vi "PLL analyzer -- PID -- V3.vi"(0 "frequency IN (Hz)":dbl=-1.0 format="%#_10f", 1 "voltage IN (V)":cdb=-0.0017981943418797428+0.0018232090265536353i format="%#_10f", 4 "time in (sec)":dbl=289.5873590533738, 5 "lorentzian IN":T2={"A (VHz)"=0.003914650866681924, "f (Hz)"=44855.11779996251, "G (Hz)"=2.9247633391664567, "phi(rad)"=3.909694945239435, "Q"=15336.32386569301, "Norm  Ampl"=nan, "bg (V)"=0.00013625172364348747-0.00019483842623467182i, "4corners"={"z (-pi/2)"=-0.0017563199699203156-0.00016210148449623068i, "z(inf)"=0.00013625172364348747-0.00019483842623467182i, "z (pi/2)"=0.0001689886653819286+0.0016977332673291314i, "z center"=-0.0007936656522691936+0.0007678158914164503i, "z(0)"=-0.0017235830281818747+0.0017304702090675725i, "radius"=0.0013384504702515796}} {"bg (V)" format="%#9_9f"; "Q" format="%#9_9f"; "phi(rad)" format="%#9_9f"; "G (Hz)" format="%#9_9f"; "f (Hz)" format="%#9_9f"}, 6 "PID action":T4, 7 "requested size":i32=100, 10 "PLL limits (Hz)":dbl=5000.0 format="%#.2f", 11 "PID mode":T1, 12 "dt (sec)":dbl=0.02 format="%#_10f", 13 "PID parameters":T5={"I (sec)"=4.747474747474747, "P (sec)"=2.0765656565656565} {"P (sec)" scale=0.01..10.0; "I (sec)" scale=0.01..10.0}) -> (14 "frequency OUT (Hz)":dbl=-1.0 format="%#_10f", 15 "overlimit ?":bool=TRUE, 18 "time out (sec)":dbl=289.5873590533738, 19 "lorentzian  OUT":T2={"A (VHz)"=0.003914650866681924, "f (Hz)"=44855.11779996251, "G (Hz)"=2.9247633391664567, "phi(rad)"=3.909694945239435, "Q"=15336.32386569301, "Norm  Ampl"=nan, "bg (V)"=0.00013625172364348747-0.00019483842623467182i, "4corners"={"z (-pi/2)"=-0.0017563199699203156-0.00016210148449623068i, "z(inf)"=0.00013625172364348747-0.00019483842623467182i, "z (pi/2)"=0.0001689886653819286+0.0016977332673291314i, "z center"=-0.0007936656522691936+0.0007678158914164503i, "z(0)"=-0.0017235830281818747+0.0017304702090675725i, "radius"=0.0013384504702515796}} {"bg (V)" format="%#9_9f"; "Q" format="%#9_9f"; "phi(rad)" format="%#9_9f"; "G (Hz)" format="%#9_9f"; "f (Hz)" format="%#9_9f"})   [LabVIEW 2020]
uses:
  pid -- parameters.ctl
  PID action.ctl
  lorentzian.ctl
  circle corners.ctl
  PID - mode.ctl
  agregator -- action.ctl
  four-corner circle transformation.ctl
  Q - not nan -- real.vi
  linear interpolation iiii- complex.vi
  linear interpolation - real.vi
panel:
  out "Plot: complex plane":cluster{dbl[], dbl[]}[](graph)=[{[], []}, {[nan, nan, nan, nan, nan, nan, nan, nan, nan, nan, nan, nan, nan, nan, nan, nan, nan, nan, nan, nan, nan, nan, nan, nan, nan, nan, nan, nan, nan, nan, nan, nan, nan, nan, nan, nan, nan, nan, nan, nan, nan, nan, nan, nan, nan, nan, nan, nan, nan, nan], [nan, nan, nan, nan, nan, nan, nan, nan, nan, nan, nan, nan, nan, nan, nan, nan, nan, nan, nan, nan, nan, nan, nan, nan, nan, nan, nan, nan, nan, nan, nan, nan, nan, nan, nan, nan, nan, nan, nan, nan, nan, nan, nan, nan, nan, nan, nan, nan, nan, nan]}, {[nan, nan, nan, nan, nan, nan, nan, nan, nan, nan, nan, nan, nan, nan, nan, nan, nan, nan, nan, nan], [nan, nan, nan, nan, nan, nan, nan, nan, nan, nan, nan, nan, nan, nan, nan, nan, nan, nan, nan, nan]}, {[nan, nan, nan, nan, nan, nan, nan, nan, nan, nan, nan, nan, nan, nan, nan, nan, nan, nan, nan, nan], [nan, nan, nan, nan, nan, nan, nan, nan, nan, nan, nan, nan, nan, nan, nan, nan, nan, nan, nan, nan]}, {[nan, nan, nan, nan, nan, nan, nan, nan, nan, nan, nan, nan, nan, nan, nan, nan, nan, nan, nan, nan], [nan, nan, nan, nan, nan, nan, nan, nan, nan, nan, nan, nan, nan, nan, nan, nan, nan, nan, nan, nan]}, {[nan, nan, nan, nan, nan, nan, nan, nan, nan, nan, nan, nan, nan, nan, nan, nan, nan, nan, nan, nan], [nan, nan, nan, nan, nan, nan, nan, nan, nan, nan, nan, nan, nan, nan, nan, nan, nan, nan, nan, nan]}, {[], []}]
  in  "Plot: complex plane - filter":cluster{dbl[], dbl[]}[](graph)=[{[], []}, {[], []}, {[0.0, 0.0, 0.0, 0.0, 0.0, 0.0, 0.0, 0.0, 0.0, 0.0, 0.0, 0.0, 0.0, 0.0, 0.0, 0.0, 0.0, 0.0, 0.0, 0.0, 0.0, 0.0, 0.0, 0.0, 0.0, 0.0, 0.0, 0.0, 0.0, 0.0, 0.0, 0.0, 0.0, 0.0, 0.0, 0.0, 0.0, 0.0, 0.0, 0.0, 0.0, 0.0, 0.0, 0.0, 0.0, 0.0, 0.0, 0.0, 0.0, 0.0, 0.0, 0.0, 0.0, 0.0, 0.0, 0.0, 0.0, 0.0, 0.0, 0.0, 0.0, 0.0, 0.0, 0.0, 0.0, 0.0, 0.0, 0.0, 0.0, 0.0, 0.0, 0.0, 0.0, 0.0, 0.0, 0.0, 0.0, 0.0, 0.0, 0.0, 0.0, 0.0, 0.0, 0.0, 0.0, 0.0, 0.0, 0.0, 0.0, 0.0, 0.0, 0.0, 0.0, 0.0, 0.0, 0.0, 0.0, 0.0, 0.0, 0.0], [0.0, 0.0, 0.0, 0.0, 0.0, 0.0, 0.0, 0.0, 0.0, 0.0, 0.0, 0.0, 0.0, 0.0, 0.0, 0.0, 0.0, 0.0, 0.0, 0.0, 0.0, 0.0, 0.0, 0.0, 0.0, 0.0, 0.0, 0.0, 0.0, 0.0, 0.0, 0.0, 0.0, 0.0, 0.0, 0.0, 0.0, 0.0, 0.0, 0.0, 0.0, 0.0, 0.0, 0.0, 0.0, 0.0, 0.0, 0.0, 0.0, 0.0, 0.0, 0.0, 0.0, 0.0, 0.0, 0.0, 0.0, 0.0, 0.0, 0.0, 0.0, 0.0, 0.0, 0.0, 0.0, 0.0, 0.0, 0.0, 0.0, 0.0, 0.0, 0.0, 0.0, 0.0, 0.0, 0.0, 0.0, 0.0, 0.0, 0.0, 0.0, 0.0, 0.0, 0.0, 0.0, 0.0, 0.0, 0.0, 0.0, 0.0, 0.0, 0.0, 0.0, 0.0, 0.0, 0.0, 0.0, 0.0, 0.0, 0.0]}, {[0.0, 0.0, 0.0], [0.0, 0.0, 0.0]}, {[nan, nan, nan, nan, nan, nan, nan, nan, nan, nan, nan, nan, nan, nan, nan, nan, nan, nan, nan, nan], [nan, nan, nan, nan, nan, nan, nan, nan, nan, nan, nan, nan, nan, nan, nan, nan, nan, nan, nan, nan]}, {[0.0, 0.0, 0.0, 0.0, 0.0, 0.0, 0.0, 0.0, 0.0, 0.0, 0.0, 0.0, 0.0, 0.0, 0.0, 0.0, 0.0, 0.0, 0.0, 0.0], [0.0, 0.0, 0.0, 0.0, 0.0, 0.0, 0.0, 0.0, 0.0, 0.0, 0.0, 0.0, 0.0, 0.0, 0.0, 0.0, 0.0, 0.0, 0.0, 0.0]}]
  out "pm lorentzian":T2={"A (VHz)"=nan, "f (Hz)"=0.0, "G (Hz)"=0.0, "phi(rad)"=nan, "Q"=nan, "Norm  Ampl"=nan, "bg (V)"=nan+nani, "4corners"={"z (-pi/2)"=nan+nani, "z(inf)"=nan+nani, "z (pi/2)"=nan+nani, "z center"=nan+nani, "z(0)"=nan+nani, "radius"=nan}} {"bg (V)" format="%#9_9f"; "Q" format="%#9_9f"; "phi(rad)" format="%#9_9f"; "G (Hz)" format="%#9_9f"; "f (Hz)" format="%#9_9f"}
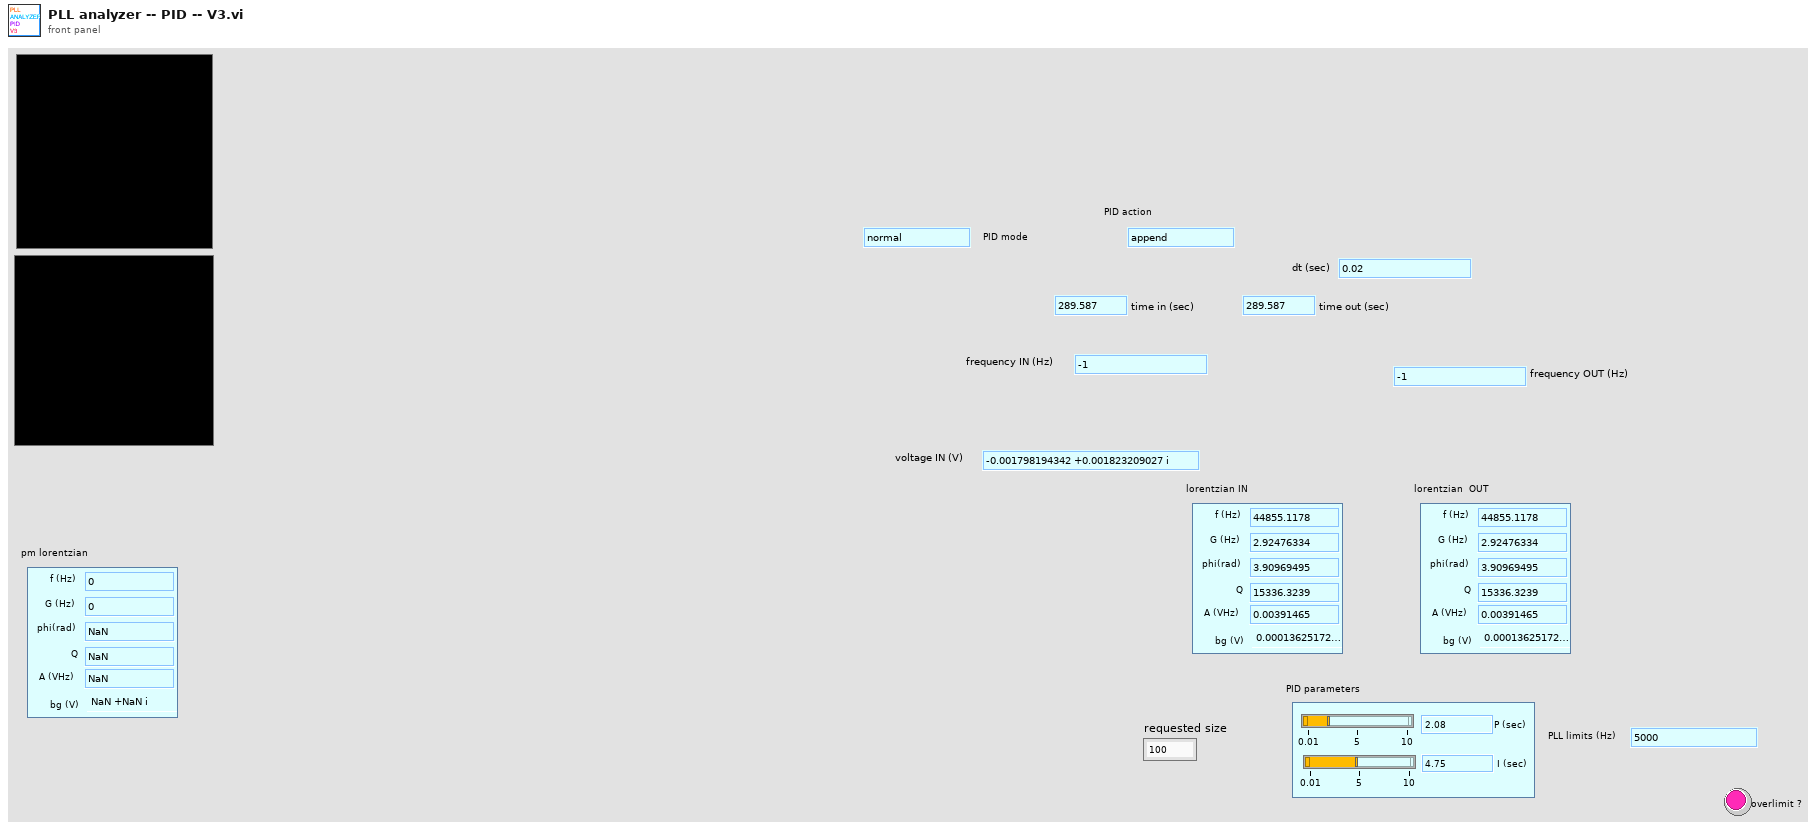
[diagram p1: front panel]
types:
  T1 = typedef "PID - mode.ctl" = enum16{"normal", "heat"}
  T2 = typedef "lorentzian.ctl" = cluster{"A (VHz)":dbl, "f (Hz)":dbl, "G (Hz)":dbl, "phi(rad)":dbl, "Q":dbl, "Norm  Ampl":dbl, "bg (V)":cdb, "4corners":T3}
  T3 = typedef "circle corners.ctl" = cluster{"z (-pi/2)":cdb, "z(inf)":cdb, "z (pi/2)":cdb, "z center":cdb, "z(0)":cdb, "radius":dbl}
  T4 = typedef "PID action.ctl" = enum16{"append", "empty!", "reset frequency", "reset from num", "overlimit"}
  T5 = typedef "pid -- parameters.ctl" = cluster{"I (sec)":dbl, "P (sec)":dbl}
  T6 = typedef "agregator -- action.ctl" = enum16{"append", "interpolate", "empty!", "force", "init", "scale", "read last"}
  T7 = typedef "four-corner circle transformation.ctl" = enum16{"z(c) z(inf)", "z(c) z(zero)", "fix phase", "calculate lorentzian", "z(0) z(+-pi/2)", "shift to zcenter", "to  canonical", "get canonical phase", "get4corners", "update lorentzian -- from z0", "fake gamma normal", "fake gamma heat", "calculate complex slope"}
  T8 = typedef "interpolation state - real.ctl" = cluster{"requested size":i32, "Array":dbl[], "actual number of elements":i32}
  T9 = typedef "interpolation state - complex.ctl" = cluster{"requested size":i32, "Array":cdb[], "actual number of elements":i32}
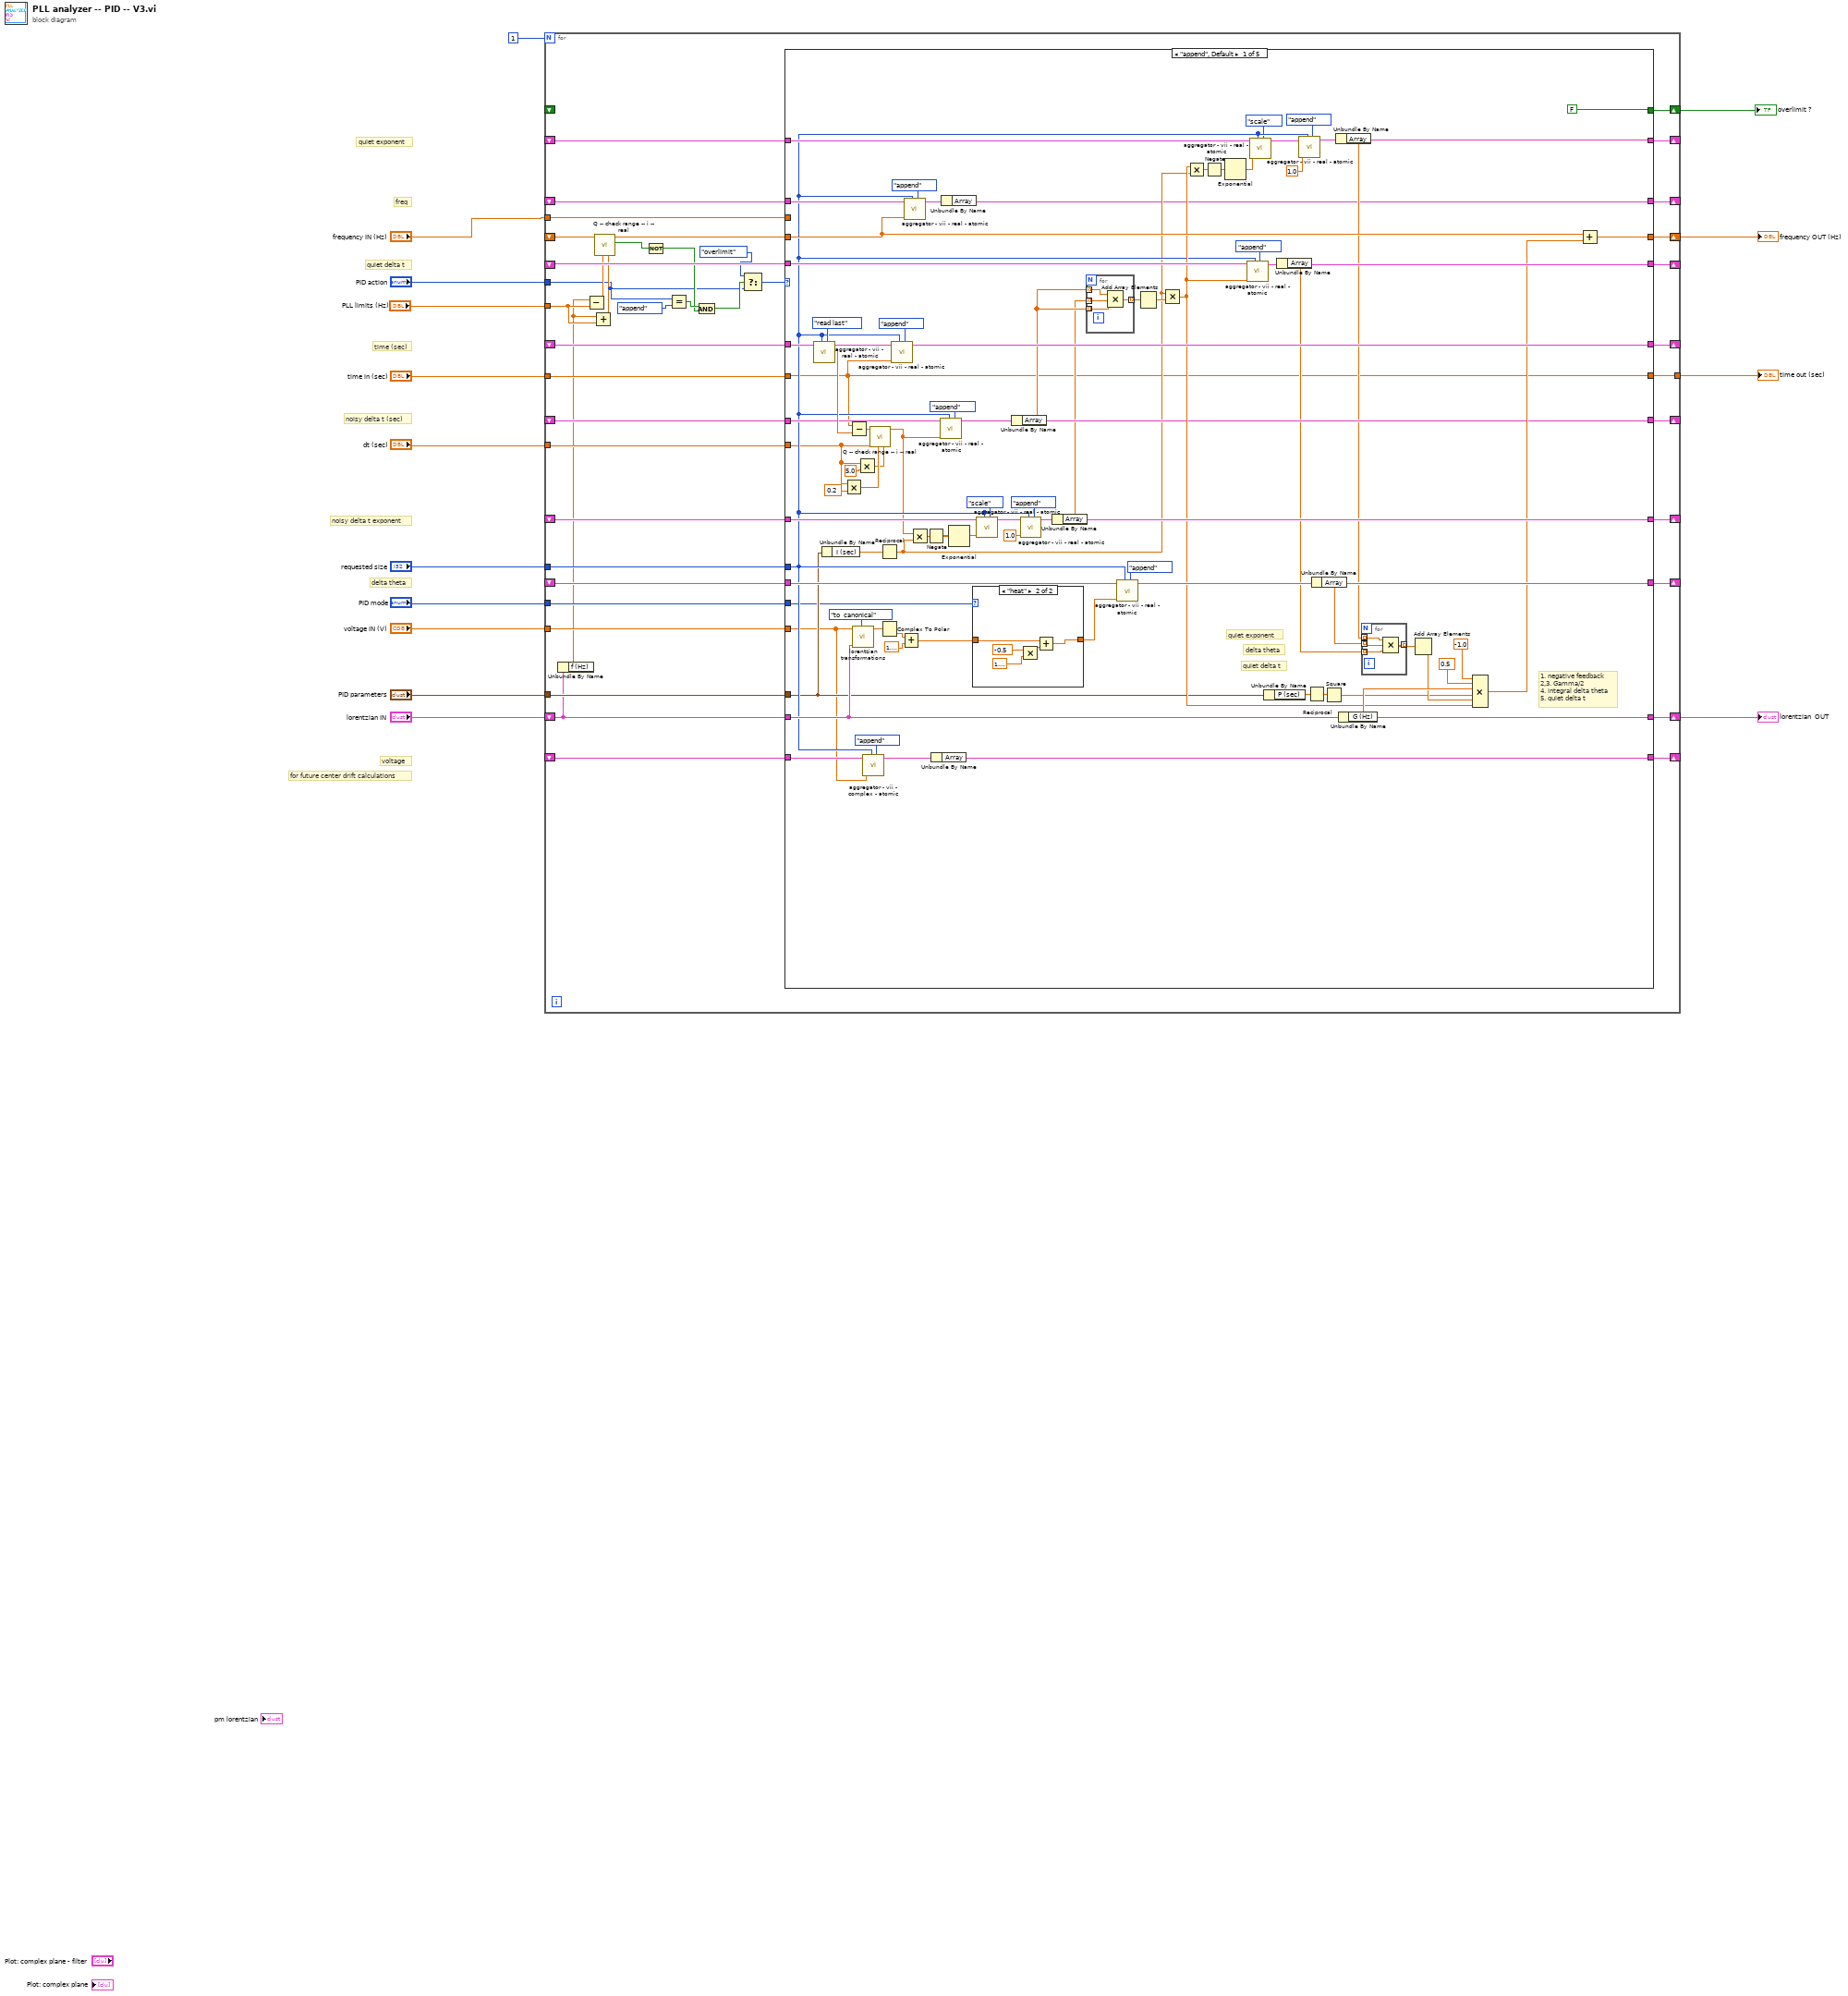
[diagram p0: block diagram]
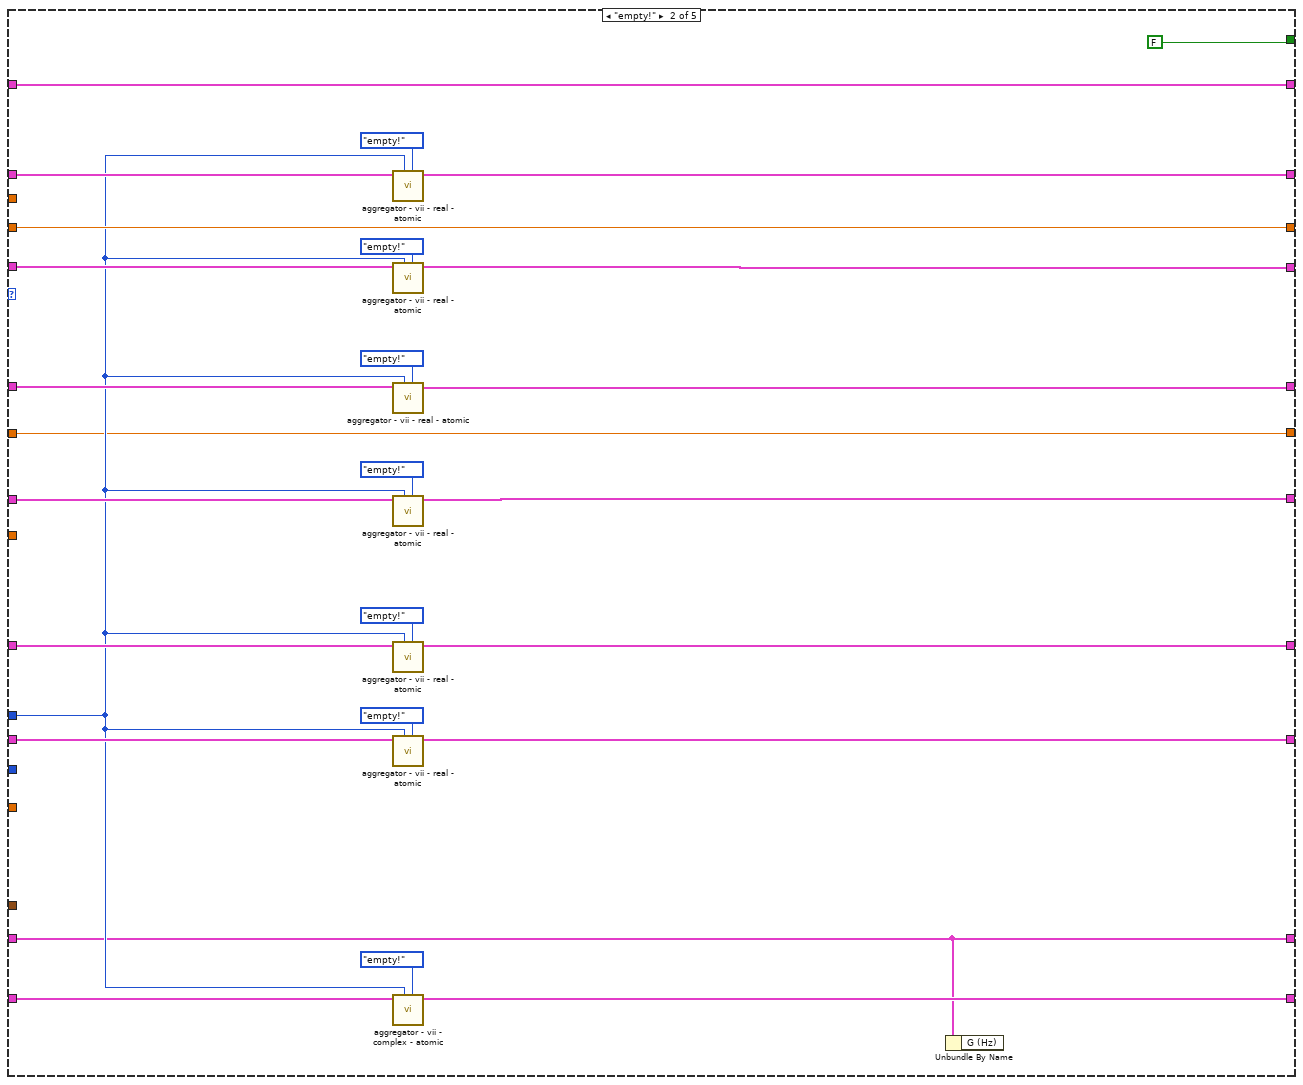
[diagram p3: hidden frame]
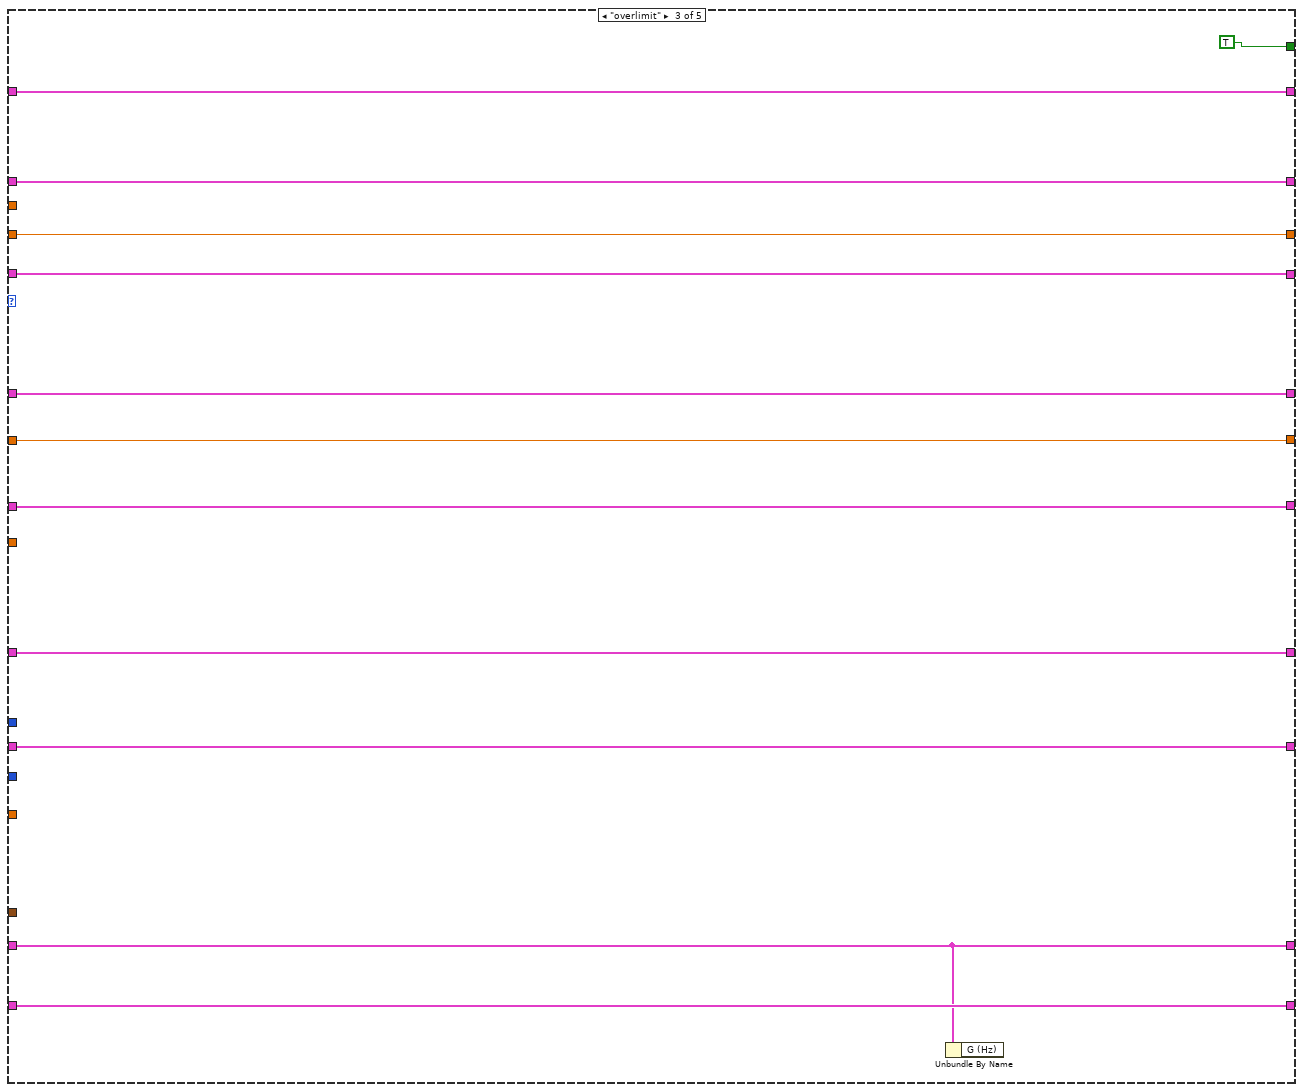
[diagram p4: hidden frame]
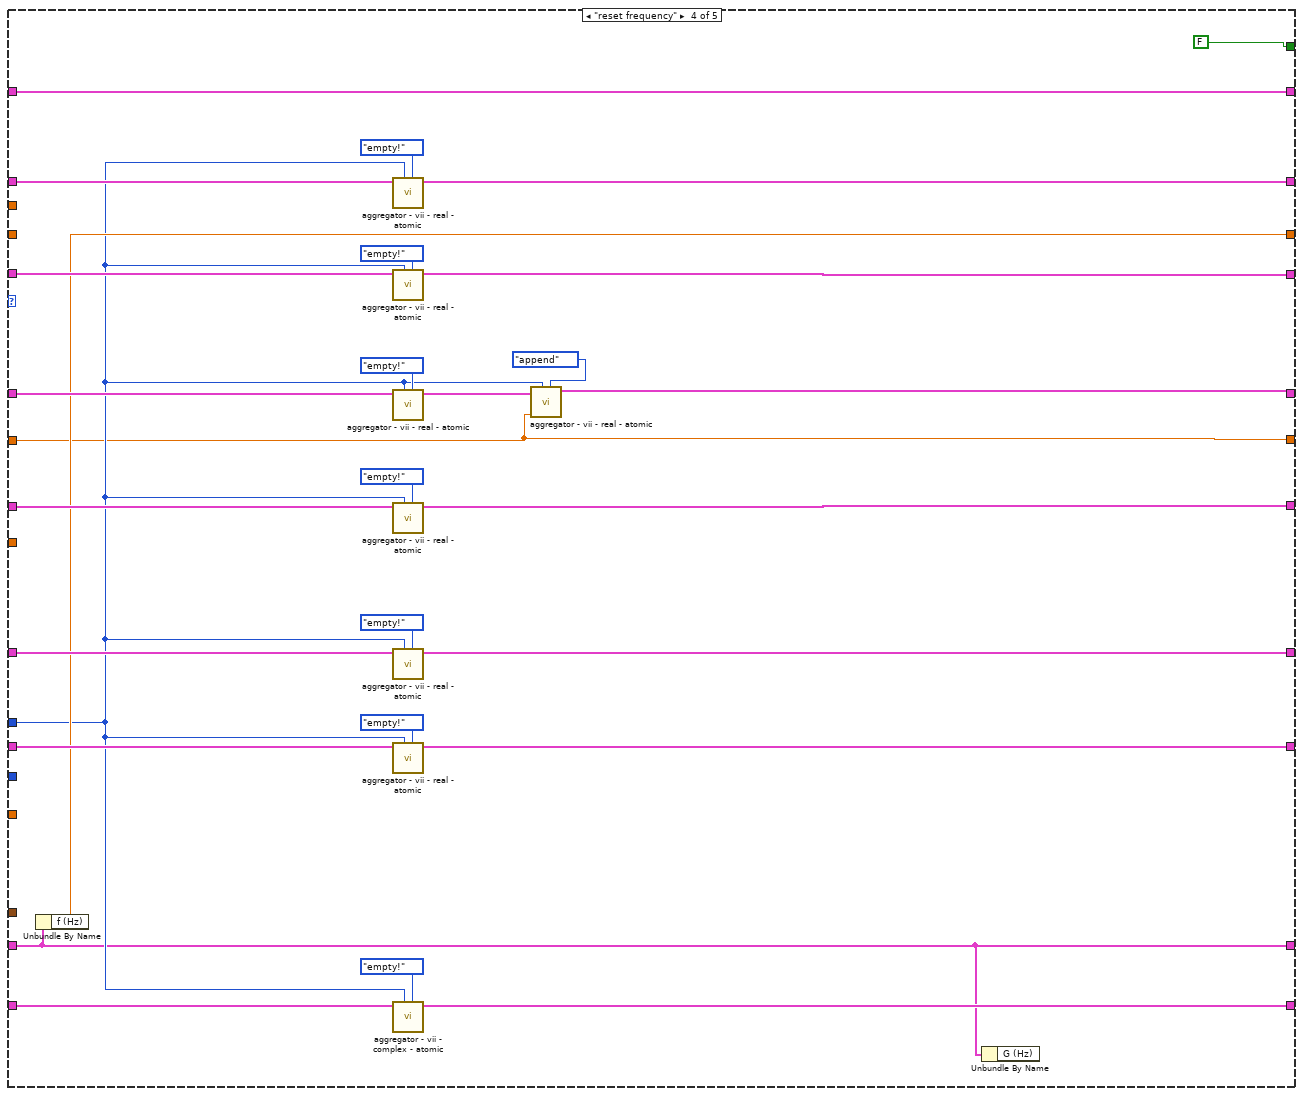
[diagram p5: hidden frame]
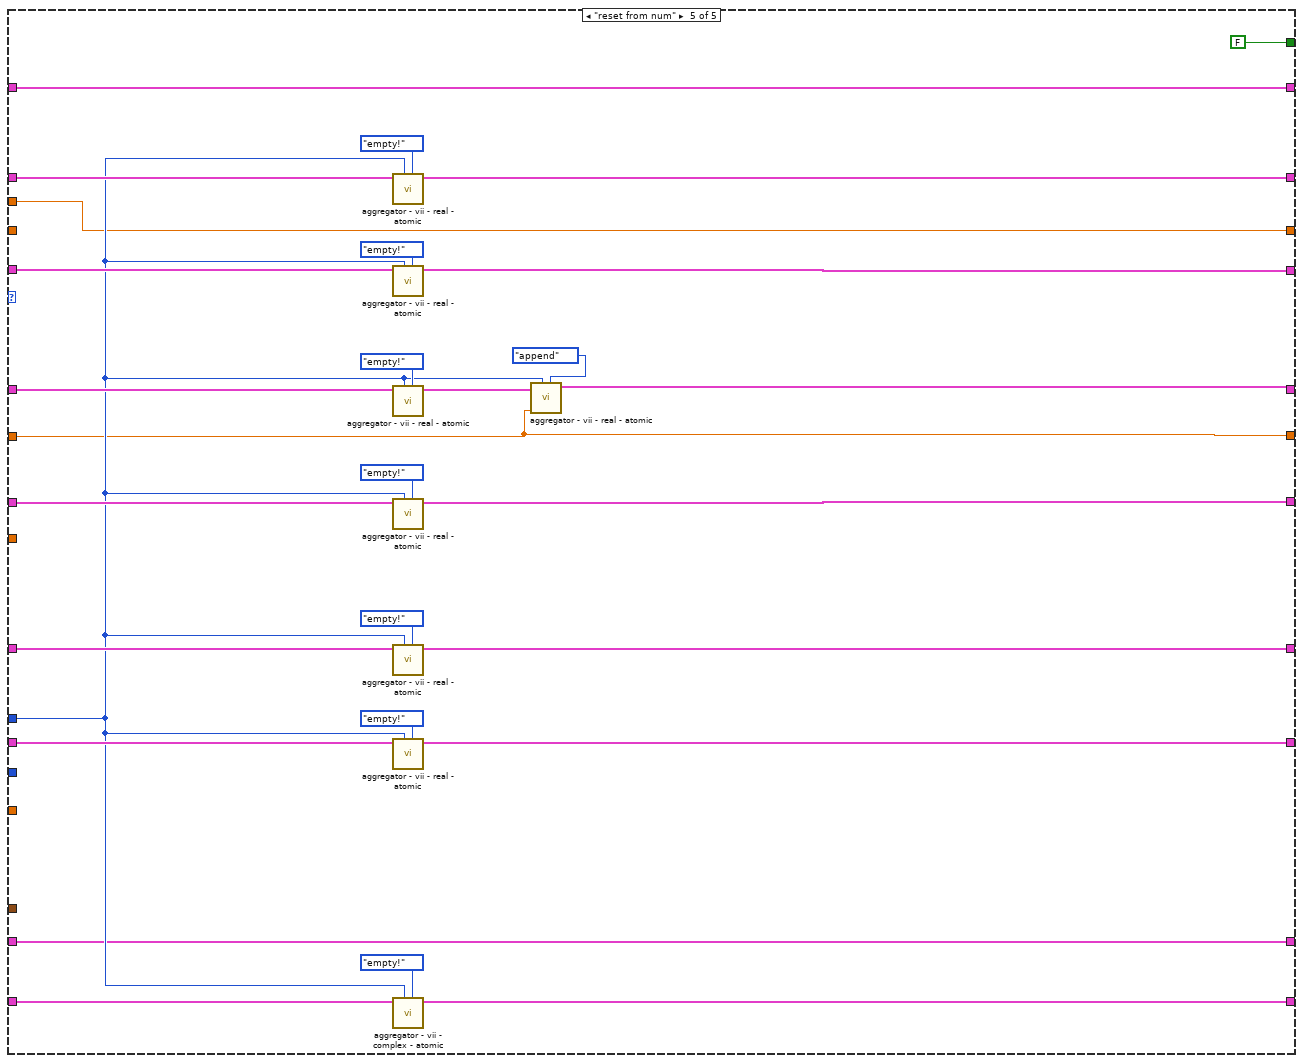
[diagram p6: hidden frame]
diagram:
  # "quiet exponent"
  # "noisy delta t exponent"
  # "for future center drift calculations"
  # "voltage"
  # "freq"
  # "delta theta"
  # "quiet delta t"
  # "time (sec)"
  # "noisy delta t (sec)"
  n1 = for {
    N: 1 -> [_]
    tunnel: "requested size" -> [w57]
    tunnel: "PID action" -> [w16]
    shift-right: [w55] -> _
    shift-left: _ -> [w56]
    tunnel: "time in (sec)" -> [w54]
    shift-right: [w52] -> _
    shift-left: _ -> [w53]
    tunnel: "voltage IN (V)" -> [w51]
    shift-right: [w49] -> _
    shift-left: _ -> [w50]
    shift-right: [w47] -> _
    shift-left: _ -> [w48]
    shift-right: [w46] -> w4
    shift-left: _ -> [w26]
    shift-right: [w45] -> w10
    shift-left: "lorentzian IN" -> [w28]
    shift-right: [w44] -> _
    shift-left: _ -> [w43]
    shift-right: [w42] -> _
    shift-left: _ -> [w41]
    shift-right: [w40] -> _
    shift-left: _ -> [w39]
    shift-right: [w38] -> _
    shift-left: _ -> [w37]
    tunnel: "frequency IN (Hz)" -> [w36]
    tunnel: "dt (sec)" -> [w35]
    tunnel: "PID parameters" -> [w34]
    tunnel: [w33] -> w6
    tunnel: "PID mode" -> [w32]
    tunnel: "PLL limits (Hz)" -> [w29]
    shift-right: [w23] -> w2
    shift-left: _ -> [_]
    n2 = Unbundle By Name(w28) -> ("f (Hz)"=w27:dbl)
    n3 = Subtract(x=w27, y=w29) -> (x-y=w31:dbl)
    n4 = Add(x=w27, y=w29) -> (x+y=w30:dbl)
    n5 = call "Q -- check range -- i -- real.vi"("upper"=w30, "lower"=w31, "number"=w26) -> ("in range?"=w20:bool, "number in range"=w25:dbl)  [unwired: 6 in, 1 out]
    n6 = Not(x=w20) -> (.not. x?=w19:bool)
    n7 = Equal?(x=w16, y=PID_action."append" ("f")) -> (x = y?=w21:bool)
    n8 = And(x=w21, y=w19) -> (x .and. y?=w18:bool)
    n9 = Select(t=PID_action."overlimit" ("f"), s=w18, f=w16) -> (s? t:f=w24:T4)
    n10 = case shown="\"append\", Default" w24 {
      tunnel: w57 -> [w95 w156 _ w195 w225]
      tunnel: w56 -> [w137 w168 w187 w209 w238]
      tunnel: [w118 w155 w187 w196 w226] -> w55
      tunnel: w54 -> [w65 w154 w181 w194 w224]
      tunnel: w53 -> [w136 w172 w189 w213 w242]
      tunnel: [w123 w171 w189 w212 w241] -> w52
      tunnel: w51 -> [w62 _ _ _ _]
      tunnel: w50 -> [w103 w170 w188 w211 w240]
      tunnel: [w90 w169 w188 w210 w239] -> w49
      tunnel: w48 -> [w127 w174 w190 w215 w244]
      tunnel: [w125 w173 w190 w214 w243] -> w47
      tunnel: w25 -> [w108 w167 w186 _ _]
      tunnel: w28 -> [w111 w153 w180 w191 w220]
      tunnel: [w120 w167 w186 w199 w222] -> w46
      tunnel: [w111 w153 w180 w191 w220] -> w45
      tunnel: [w59 w165 w185 w193 w223] -> w44
      tunnel: w43 -> [w110 w166 w185 w208 w237]
      tunnel: [w58 w161 w184 w204 w233] -> w42
      tunnel: w41 -> [w109 w162 w184 w205 w234]
      tunnel: [w92 w159 w183 w202 w231] -> w40
      tunnel: w39 -> [w100 w158 w183 w201 w230]
      tunnel: [w91 w157 w182 w200 w229] -> w38
      tunnel: w37 -> [w99 w157 w182 w200 w229]
      tunnel: w36 -> [_ _ _ _ w222]
      tunnel: w35 -> [w75 _ _ _ _]
      tunnel: w34 -> [w68 _ _ _ _]
      tunnel: [w65 w154 w181 w194 w224] -> w33
      tunnel: w32 -> [w61 _ _ _ _]
      tunnel: [FALSE FALSE TRUE FALSE FALSE] -> w23
      frame "append", Default {
        # "1. negative feedback\n2,3. Gamma/2\n4. integral delta theta\n5. quiet delta t"
        # "quiet delta t"
        # "delta theta"
        # "quiet exponent"
        n11 = call "aggregator - vii - real - atomic.vi"("aggregator action"=agregator_--_action."read last", "requested size"=w95, "state IN"=w137) -> ("mean"=w130:dbl, "state OUT"=w119:T8)  [unwired: 5 in, 2 out]
        n12 = Unbundle By Name(w68) -> ("I (sec)"=w67:dbl)
        n13 = Multiply(x=w75, y=0.2 ("upper")) -> (x*y=w81:dbl)
        n14 = Subtract(x=w65, y=w130) -> (x-y=w85:dbl)
        n15 = call "lorentzian transformations.vi"("4 corner circle transformation"=four-corner_circle_transformation."to  canonical", "lorentzian in"=w111, "voltage in"=w62) -> ("voltage out"=w115:cdb)  [unwired: 5 in, 3 out]
        n16 = Multiply(x=w75, y=5.0 ("upper")) -> (x*y=w73:dbl)
        n17 = call "aggregator - vii - complex - atomic.vi"("aggregator action"=agregator_--_action."append", "requested size"=w95, "number"=w62, "state IN"=w110) -> ("state OUT"=w59:T9)  [unwired: 4 in, 3 out]
        n18 = call "Q -- check range -- i -- real.vi"("upper"=w73, "lower"=w81, "default"=w75, "number"=w85) -> ("number in range"=w83:dbl)  [unwired: 5 in, 2 out]
        n19 = Reciprocal(x=w67) -> (1/x=w66:dbl)
        n20 = Complex To Polar(r * e^(i*theta)=w115) -> (theta=w114:dbl)  [unwired: 1 out]
        n21 = call "aggregator - vii - real - atomic.vi"("aggregator action"=agregator_--_action."append", "requested size"=w95, "number"=w65, "state IN"=w119) -> ("state OUT"=w118:T8)  [unwired: 4 in, 3 out]
        n22 = Add(x=w114, y=1.5707963267948966) -> (x+y=w64:dbl)
        n23 = call "aggregator - vii - real - atomic.vi"("aggregator action"=agregator_--_action."append", "requested size"=w95, "number"=w108, "state IN"=w109) -> ("state OUT"=w58:T8)  [unwired: 4 in, 3 out]
        n24 = Multiply(x=w83, y=w66) -> (x*y=w87:dbl)
        n25 = Negate(x=w87) -> (-x=w84:dbl)
        n26 = Unbundle By Name(w59) -> ()  [unwired: 1 out]
        n27 = call "aggregator - vii - real - atomic.vi"("aggregator action"=agregator_--_action."append", "requested size"=w95, "number"=w83, "state IN"=w103) -> ("state OUT"=w90:T8)  [unwired: 4 in, 3 out]
        n28 = Unbundle By Name(w58) -> ()  [unwired: 1 out]
        n29 = Exponential(1:w84) -> (0:w86:dbl)
        n30 = case shown="\"heat\"" w61 {
          tunnel: w64 -> [w138 w143]
          tunnel: [w138 w142] -> w63
          frame "normal", Default {
          }
          frame "heat" {
            n31 = Multiply(x=-0.5, y=1.5707963267948966) -> (x*y=w139:dbl)
            n32 = Add(x=w143, y=w139) -> (x+y=w142:dbl)
          }
        }
        n33 = call "aggregator - vii - real - atomic.vi"("aggregator action"=agregator_--_action."scale", "requested size"=w95, "number"=w86, "state IN"=w136) -> ("state OUT"=w135:T8)  [unwired: 4 in, 3 out]
        n34 = Unbundle By Name(w90) -> ("Array"=w102:dbl[])
        n35 = call "aggregator - vii - real - atomic.vi"("aggregator action"=agregator_--_action."append", "requested size"=w95, "number"=1.0, "state IN"=w135) -> ("state OUT"=w123:T8)  [unwired: 4 in, 3 out]
        n36 = Unbundle By Name(w123) -> ("Array"=w89:dbl[])
        n37 = for {
          tunnel: [w147] -> w104 mode=indexing
          tunnel: w102 -> [w146] mode=indexing
          tunnel: w89 -> [w145] mode=indexing
          tunnel: w102 -> [w144] mode=indexing
          n38 = Compound Arithmetic op=MULTIPLY(w146, w145, w144) -> (w147:dbl)
        }
        n39 = call "aggregator - vii - real - atomic.vi"("aggregator action"=agregator_--_action."append", "requested size"=w95, "number"=w63, "state IN"=w127) -> ("state OUT"=w125:T8)  [unwired: 4 in, 3 out]
        n40 = Add Array Elements(numeric array=w104) -> (sum=w74:dbl)
        n41 = Multiply(x=w66, y=w74) -> (x*y=w98:dbl)
        n42 = Multiply(x=w98, y=w66) -> (x*y=w78:dbl)
        n43 = Negate(x=w78) -> (-x=w77:dbl)
        n44 = Exponential(1:w77) -> (0:w76:dbl)
        n45 = call "aggregator - vii - real - atomic.vi"("aggregator action"=agregator_--_action."append", "requested size"=w95, "number"=w98, "state IN"=w100) -> ("state OUT"=w92:T8)  [unwired: 4 in, 3 out]
        n46 = call "aggregator - vii - real - atomic.vi"("aggregator action"=agregator_--_action."scale", "requested size"=w95, "number"=w76, "state IN"=w99) -> ("state OUT"=w97:T8)  [unwired: 4 in, 3 out]
        n47 = Unbundle By Name(w68) -> ("P (sec)"=w71:dbl)
        n48 = Unbundle By Name(w92) -> ("Array"=w80:dbl[])
        n49 = call "aggregator - vii - real - atomic.vi"("aggregator action"=agregator_--_action."append", "requested size"=w95, "number"=1.0, "state IN"=w97) -> ("state OUT"=w91:T8)  [unwired: 4 in, 3 out]
        n50 = Reciprocal(x=w71) -> (1/x=w70:dbl)
        n51 = Unbundle By Name(w125) -> ("Array"=w88:dbl[])
        n52 = Square(x=w70) -> (x^2=w69:dbl)
        n53 = Unbundle By Name(w91) -> ("Array"=w79:dbl[])
        n54 = Unbundle By Name(w111) -> ("G (Hz)"=w122:dbl)
        n55 = for {
          tunnel: w88 -> [w151] mode=indexing
          tunnel: [w150] -> w124 mode=indexing
          tunnel: w80 -> [w149] mode=indexing
          tunnel: w79 -> [w148] mode=indexing
          n56 = Compound Arithmetic op=MULTIPLY(w148, w151, w149) -> (w150:dbl)
        }
        n57 = Add Array Elements(numeric array=w124) -> (sum=w121:dbl)
        n58 = Compound Arithmetic op=MULTIPLY(-1.0 ("value"), 0.5 ("value"), w122, w69, w121, w98) -> (w105:dbl)
        n59 = Add(x=w108, y=w105) -> (x+y=w120:dbl)
      }
      frame "empty!" {
        n60 = call "aggregator - vii - real - atomic.vi"("aggregator action"=agregator_--_action."empty!", "requested size"=w156, "state IN"=w162) -> ("state OUT"=w161:T8)  [unwired: 5 in, 3 out]
        n61 = call "aggregator - vii - real - atomic.vi"("aggregator action"=agregator_--_action."empty!", "requested size"=w156, "state IN"=w158) -> ("state OUT"=w159:T8)  [unwired: 5 in, 3 out]
        n62 = call "aggregator - vii - real - atomic.vi"("aggregator action"=agregator_--_action."empty!", "requested size"=w156, "state IN"=w168) -> ("state OUT"=w155:T8)  [unwired: 5 in, 3 out]
        n63 = call "aggregator - vii - real - atomic.vi"("aggregator action"=agregator_--_action."empty!", "requested size"=w156, "state IN"=w170) -> ("state OUT"=w169:T8)  [unwired: 5 in, 3 out]
        n64 = call "aggregator - vii - real - atomic.vi"("aggregator action"=agregator_--_action."empty!", "requested size"=w156, "state IN"=w172) -> ("state OUT"=w171:T8)  [unwired: 5 in, 3 out]
        n65 = call "aggregator - vii - real - atomic.vi"("aggregator action"=agregator_--_action."empty!", "requested size"=w156, "state IN"=w174) -> ("state OUT"=w173:T8)  [unwired: 5 in, 3 out]
        n66 = call "aggregator - vii - complex - atomic.vi"("aggregator action"=agregator_--_action."empty!", "requested size"=w156, "state IN"=w166) -> ("state OUT"=w165:T9)  [unwired: 5 in, 3 out]
        n67 = Unbundle By Name(w153) -> ()  [unwired: 1 out]
      }
      frame "overlimit" {
        n68 = Unbundle By Name(w180) -> ()  [unwired: 1 out]
      }
      frame "reset frequency" {
        n69 = Unbundle By Name(w191) -> ("f (Hz)"=w199:dbl)
        n70 = call "aggregator - vii - real - atomic.vi"("aggregator action"=agregator_--_action."empty!", "requested size"=w195, "state IN"=w205) -> ("state OUT"=w204:T8)  [unwired: 5 in, 3 out]
        n71 = call "aggregator - vii - real - atomic.vi"("aggregator action"=agregator_--_action."empty!", "requested size"=w195, "state IN"=w201) -> ("state OUT"=w202:T8)  [unwired: 5 in, 3 out]
        n72 = call "aggregator - vii - real - atomic.vi"("aggregator action"=agregator_--_action."empty!", "requested size"=w195, "state IN"=w209) -> ("state OUT"=w197:T8)  [unwired: 5 in, 3 out]
        n73 = call "aggregator - vii - real - atomic.vi"("aggregator action"=agregator_--_action."empty!", "requested size"=w195, "state IN"=w211) -> ("state OUT"=w210:T8)  [unwired: 5 in, 3 out]
        n74 = call "aggregator - vii - real - atomic.vi"("aggregator action"=agregator_--_action."empty!", "requested size"=w195, "state IN"=w213) -> ("state OUT"=w212:T8)  [unwired: 5 in, 3 out]
        n75 = call "aggregator - vii - real - atomic.vi"("aggregator action"=agregator_--_action."empty!", "requested size"=w195, "state IN"=w215) -> ("state OUT"=w214:T8)  [unwired: 5 in, 3 out]
        n76 = call "aggregator - vii - complex - atomic.vi"("aggregator action"=agregator_--_action."empty!", "requested size"=w195, "state IN"=w208) -> ("state OUT"=w193:T9)  [unwired: 5 in, 3 out]
        n77 = call "aggregator - vii - real - atomic.vi"("aggregator action"=agregator_--_action."append", "requested size"=w195, "number"=w194, "state IN"=w197) -> ("state OUT"=w196:T8)  [unwired: 4 in, 3 out]
        n78 = Unbundle By Name(w191) -> ()  [unwired: 1 out]
      }
      frame "reset from num" {
        n79 = call "aggregator - vii - real - atomic.vi"("aggregator action"=agregator_--_action."empty!", "requested size"=w225, "state IN"=w234) -> ("state OUT"=w233:T8)  [unwired: 5 in, 3 out]
        n80 = call "aggregator - vii - real - atomic.vi"("aggregator action"=agregator_--_action."empty!", "requested size"=w225, "state IN"=w230) -> ("state OUT"=w231:T8)  [unwired: 5 in, 3 out]
        n81 = call "aggregator - vii - real - atomic.vi"("aggregator action"=agregator_--_action."empty!", "requested size"=w225, "state IN"=w238) -> ("state OUT"=w227:T8)  [unwired: 5 in, 3 out]
        n82 = call "aggregator - vii - real - atomic.vi"("aggregator action"=agregator_--_action."empty!", "requested size"=w225, "state IN"=w240) -> ("state OUT"=w239:T8)  [unwired: 5 in, 3 out]
        n83 = call "aggregator - vii - real - atomic.vi"("aggregator action"=agregator_--_action."empty!", "requested size"=w225, "state IN"=w242) -> ("state OUT"=w241:T8)  [unwired: 5 in, 3 out]
        n84 = call "aggregator - vii - real - atomic.vi"("aggregator action"=agregator_--_action."empty!", "requested size"=w225, "state IN"=w244) -> ("state OUT"=w243:T8)  [unwired: 5 in, 3 out]
        n85 = call "aggregator - vii - complex - atomic.vi"("aggregator action"=agregator_--_action."empty!", "requested size"=w225, "state IN"=w237) -> ("state OUT"=w223:T9)  [unwired: 5 in, 3 out]
        n86 = call "aggregator - vii - real - atomic.vi"("aggregator action"=agregator_--_action."append", "requested size"=w225, "number"=w224, "state IN"=w227) -> ("state OUT"=w226:T8)  [unwired: 4 in, 3 out]
      }
    }
  }
  "lorentzian  OUT" <- w10
  "time out (sec)" <- w6
  "frequency OUT (Hz)" <- w4
  "overlimit ?" <- w2
